vi "Cannon Logic.vi"() -> ()   [LabVIEW 2019]
uses:
  <vilib>/Rock Robotics/WPI/Solenoid/WPI_SolenoidValue.ctl
  <vilib>/Rock Robotics/WPI/ThirdParty/Phoenix-LabVIEW/Motor Controller/Controls/CTRE_Phoenix_MotorControl_ControlMode.ctl
  <vilib>/Rock Robotics/Network Tables/NT Read Boolean.vi
  Robot Global Data.vi
  <vilib>/Rock Robotics/WPI/Solenoid/WPI_SolenoidSetEnum.vi
panel:
  out "ballcount":i16
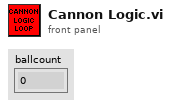
[diagram p1: front panel]
types:
  T1 = typedef "WPI_SolenoidDevRef.ctl" = cluster{"DevStatus":errorcluster, "Pneumatics Control Module":u8, "Forward Solenoid Channel":T2, "Reverse Solenoid Channel":T2}
  T2 = typedef "WPI_SolenoidChannel.ctl" = enum8{"Solenoid 0", "Solenoid 1", "Solenoid 2", "Solenoid 3", "Solenoid 4", "Solenoid 5", "Solenoid 6", "Solenoid 7", "Invalid"}
  T3 = typedef "WPI_MotorControlDeviceRef.ctl" = cluster{"DeviceStatus":errorcluster, "Type":T4, "PWM":cluster{"PWM Channel":T5, "DeadBand":T6}, "CAN":cluster{"Device Number":u8, "SetOutput VI Ref":variant, "GetOutput VI Ref":variant, "Enable VI Ref":variant, "Disable VI Ref":variant, "Data":variant}, "Invert":bool, "DIO PWM":cluster{"PWM \"Enable\" Channel":T5, "DIOChannel":T7, "PWM Rate":dbl}}
  T4 = typedef "WPI_MotorControlType.ctl" = enum16{"PWM", "CAN", "DIO PWM"}
  T5 = typedef "FPGA_DIOPWMChannel.ctl" = enum8{"PWM 0", "PWM 1", "PWM 2", "PWM 3", "PWM 4", "PWM 5", "PWM 6", "PWM 7", "PWM 8", "PWM 9", "PWM MXP 0", "PWM MXP 1", "PWM MXP 2", "PWM MXP 3", "PWM MXP 4", "PWM MXP 5", "PWM MXP 6", "PWM MXP 7", "PWM MXP 8", "PWM MXP 9", "Invalid"}
  T6 = typedef "WPI_PWMDeadband.ctl" = cluster{"Name":string, "maxPositivePwm":i32, "minPositivePwm":i32, "centerPwm":i32, "maxNegativePwm":i32, "minNegativePwm":i32, "angularRange":u16}
  T7 = typedef "FPGA_DIOChannel.ctl" = enum8{"DIO 0", "DIO 1", "DIO 2", "DIO 3", "DIO 4", "DIO 5", "DIO 6", "DIO 7", "DIO 8", "DIO 9", "DIO MXP 0", "DIO MXP 1", "DIO MXP 2", "DIO MXP 3", "DIO MXP 4", "DIO MXP 5", "DIO MXP 6", "DIO MXP 7", "DIO MXP 8", "DIO MXP 9", "DIO MXP 10", "DIO MXP 11", "DIO MXP 12", "DIO MXP 13", "DIO MXP 14", "DIO MXP 15", "SPI Port CS1", "SPI Port CS2", "SPI Port CS3", "SPI Port MISO", "SPI Port MOSI", "Invalid"}
  T8 = typedef "WPI_AnalogChannelDevRef.ctl" = cluster{"DevStatus":errorcluster, "Analog Channel":T9}
  T9 = typedef "FPGA_AIChannel.ctl" = enum8{"AI 0", "AI 1", "AI 2", "AI 3", "AI MXP 0", "AI MXP 1", "AI MXP 2", "AI MXP 3", "Invalid"}
  T10 = typedef "WPI_SolenoidValue.ctl" = enum16{"Off", "On", "Forward", "Reverse"}
  T11 = typedef "CTRE_Phoenix_MotorControl_ControlMode.ctl" = u16
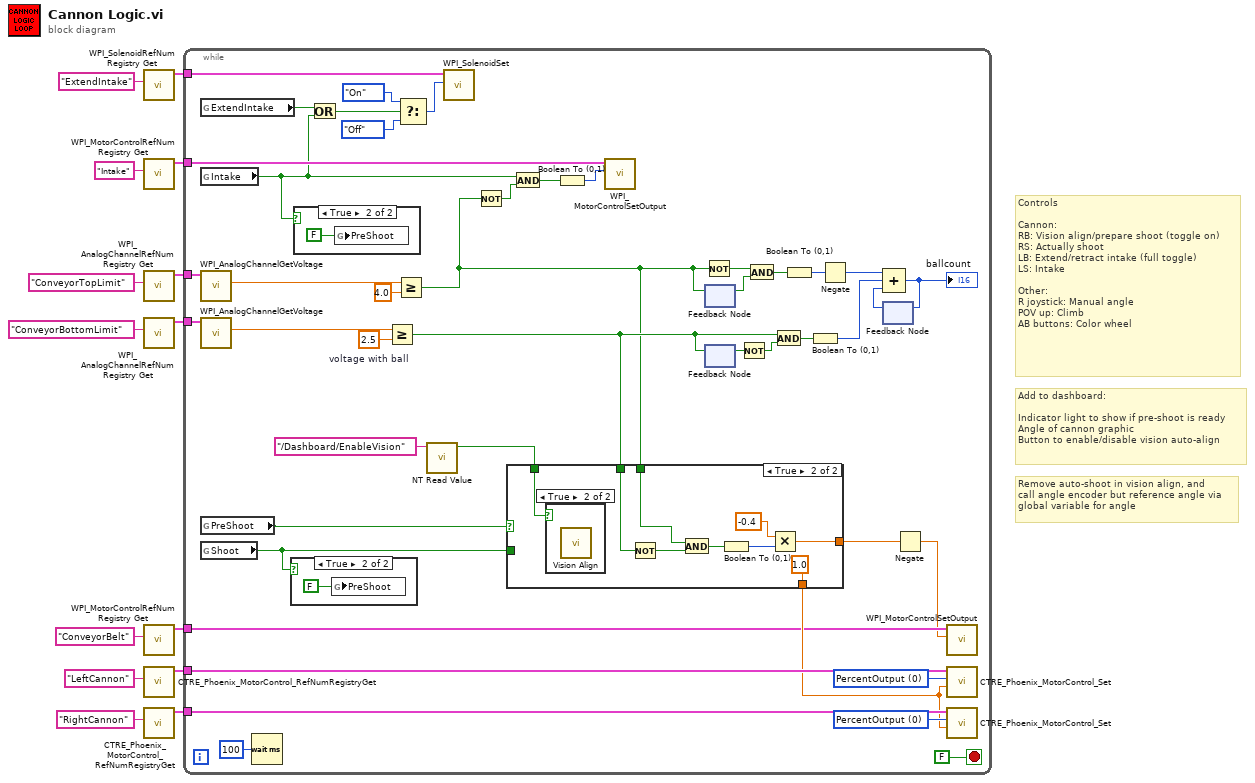
[diagram p0: block diagram]
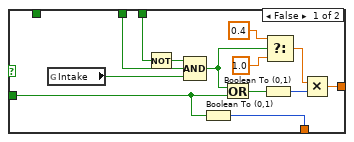
[diagram p4: hidden frame]
diagram:
  # "Remove auto-shoot in vision align, and\ncall angle encoder but reference angle via\nglobal variable for angle"
  # "Add to dashboard:\n\nIndicator light to show if pre-shoot is ready\nAngle of cannon graphic\nButton to enable/disable vision auto-align"
  # "Controls\n\nCannon:\nRB: Vision align/prepare shoot (toggle on)\nRS: Actually shoot\nLB: Extend/retract intake (full toggle)\nLS: Intake\n\nOther:\nR joystick: Manual angle\nPOV up: Climb\nAB buttons: Color wheel"
  n1 = call <vilib>:"WPI_SolenoidRefNum Registry Get.vi"("refnum name"="ExtendIntake") -> ("SolenoidDevRef"=w8:T1)  [unwired: 9 in, 1 out]
  n2 = call <vilib>:"WPI_MotorControlRefNum Registry Get.vi"("refnum name"="Intake") -> ("MotorControlDevRef"=w7:T3)  [unwired: 9 in, 1 out]
  n3 = call <vilib>:"WPI_AnalogChannelRefNum Registry Get.vi"("refnum name"="ConveyorTopLimit") -> ("AIDeviceRef"=w4:T8)  [unwired: 9 in, 1 out]
  n4 = call <vilib>:"WPI_AnalogChannelRefNum Registry Get.vi"("refnum name"="ConveyorBottomLimit") -> ("AIDeviceRef"=w5:T8)  [unwired: 9 in, 1 out]
  n5 = call <vilib>:"WPI_MotorControlRefNum Registry Get.vi"("refnum name"="ConveyorBelt") -> ("MotorControlDevRef"=w3:T3)  [unwired: 9 in, 1 out]
  n6 = call <vilib>:"CTRE_Phoenix_MotorControl_RefNumRegistryGet.vi"("refnum name"="LeftCannon") -> ("PhoenixMotorControlDevRef"=w1:T3)  [unwired: 9 in, 1 out]
  n7 = call <vilib>:"CTRE_Phoenix_MotorControl_RefNumRegistryGet.vi"("refnum name"="RightCannon") -> ("PhoenixMotorControlDevRef"=w6:T3)  [unwired: 9 in, 1 out]
  n8 = while {
    tunnel: w8 -> [w54]
    tunnel: w7 -> [w40]
    tunnel: w6 -> [w52]
    tunnel: w5 -> [w51]
    tunnel: w4 -> [w50]
    tunnel: w3 -> [w39]
    tunnel: w1 -> [w46]
    stop <- FALSE stop-if-true
    w47 = T11 0 items=["PercentOutput"=0, "Position"=1, "Velocity"=2, "Current"=3, "Follower"=5, "MotionProfile"=6, "MotionMagic"=7, "MotionProfileArc"=10, "Disabled"=15] ("Control Mode")
    w45 = T11 0 items=["PercentOutput"=0, "Position"=1, "Velocity"=2, "Current"=3, "Follower"=5, "MotionProfile"=6, "MotionMagic"=7, "MotionProfileArc"=10, "Disabled"=15] ("Control Mode")
    w48 = 2.5  # voltage with ball
    n9 = global read "Robot Global Data.vi" "ExtendIntake"() -> (w26:bool)
    n10 = global read "Robot Global Data.vi" "Intake"() -> (w19:bool)
    n11 = call <vilib>:"WPI_AnalogChannelGetVoltage.vi"("AIDeviceRef"=w50) -> ("Voltage"=w21:dbl)  [unwired: 8 in, 2 out]
    n12 = call <vilib>:"WPI_AnalogChannelGetVoltage.vi"("AIDeviceRef"=w51) -> ("Voltage"=w20:dbl)  [unwired: 8 in, 2 out]
    n13 = global read "Robot Global Data.vi" "PreShoot"() -> (w24:bool)
    n14 = global read "Robot Global Data.vi" "Shoot"() -> (w25:bool)
    n15 = Wait (ms)(milliseconds to wait=u32 100) -> ()  [unwired: 1 out]
    n16 = case shown="True" w25 {
      frame False {
      }
      frame True {
        n17 = global write "Robot Global Data.vi" "PreShoot"(FALSE ("PreShoot")) -> ()
      }
    }
    n18 = case shown="True" w19 {
      frame False {
      }
      frame True {
        n19 = global write "Robot Global Data.vi" "PreShoot"(FALSE ("PreShoot")) -> ()
      }
    }
    n20 = Or(x=w26, y=w19) -> (x .or. y?=w57:bool)
    n21 = Greater Or Equal?(x=w20, y=w48) -> (x >= y?=w16:bool)
    n22 = Greater Or Equal?(x=w21, y=4.0) -> (x >= y?=w15:bool)
    n23 = Select(t=WPI_SolenoidValue."On" ("Value"), s=w57, f=WPI_SolenoidValue."Off" ("Value")) -> (s? t:f=w53:T10)
    n24 = call-poly <vilib>:"NT Read Value.vi"("Name"="/Dashboard/EnableVision") -> ("Boolean"=w38:bool)  [unwired: 9 in, 1 out]
    n25 = call-poly <vilib>:"WPI_SolenoidSet.vi"("Value"=w53, "SolenoidDevRef"=w54) -> ()  [unwired: 8 in, 2 out]
    n26 = Not(x=w15) -> (.not. x?=w17:bool)
    n27 = case shown="True" w24 {
      tunnel: [w71 w74] -> w22
      tunnel: [w70 1.0] -> w41
      tunnel: w25 -> [w62 _]
      tunnel: w15 -> [w63 w76]
      tunnel: w38 -> [_ w82]
      tunnel: w16 -> [w72 w77]
      frame False {
        n28 = global read "Robot Global Data.vi" "Intake"() -> (w69:bool)
        n29 = Not(x=w63) -> (.not. x?=w61:bool)
        n30 = Compound Arithmetic op=AND(w61, w72, w69) -> (w67:bool)
        n31 = Boolean To (0,1)(Boolean=w62) -> (0, 1=w70:i16)
        n32 = Or(x=w67, y=w62) -> (x .or. y?=w73:bool)
        n33 = Boolean To (0,1)(Boolean=w73) -> (0, 1=w65:i16)
        n34 = Select(t=0.4, s=w67, f=1.0) -> (s? t:f=w64:dbl)
        n35 = Multiply(x=w64, y=w65) -> (x*y=w71:dbl)
      }
      frame True {
        n36 = case shown="True" w82 {
          frame False {
          }
          frame True {
            n37 = call "Vision Align.vi"() -> ()  [unwired: 12 in]
          }
        }
        n38 = Not(x=w77) -> (.not. x?=w75:bool)
        n39 = And(x=w76, y=w75) -> (x .and. y?=w79:bool)
        n40 = Boolean To (0,1)(Boolean=w79) -> (0, 1=w80:i16)
        n41 = Multiply(x=-0.4, y=w80) -> (x*y=w74:dbl)
      }
    }
    n42 = And(x=w19, y=w17) -> (x .and. y?=w18:bool)
    n43 = Boolean To (0,1)(Boolean=w18) -> (0, 1=w49:i16)
    n44 = call <vilib>:"WPI_MotorControlSetOutput.vi"("Output"=w49, "MotorControlDevRef"=w40) -> ()  [unwired: 7 in, 3 out]
    n45 = Not(x=w15) -> (.not. x?=w37:bool)
    n46 = feedback-in #1(w15) -> ()
    n47 = feedback #1() -> (w36:bool)  [unwired: 1 in]
    n48 = feedback #2() -> (w35:bool)  [unwired: 1 in]
    n49 = feedback-in #2(w16) -> ()
    n50 = Not(x=w35) -> (.not. x?=w34:bool)
    n51 = And(x=w37, y=w36) -> (x .and. y?=w33:bool)
    n52 = And(x=w16, y=w34) -> (x .and. y?=w32:bool)
    n53 = Boolean To (0,1)(Boolean=w33) -> (0, 1=w31:i16)
    n54 = Boolean To (0,1)(Boolean=w32) -> (0, 1=w27:i16)
    n55 = Negate(x=w31) -> (-x=w30:i16)
    n56 = feedback #3() -> (w29:i16)  [unwired: 1 in]
    n57 = Compound Arithmetic op=ADD(w30, w27, w29) -> (w28:i16)
    "ballcount" <- w28
    n58 = feedback-in #3(w28) -> ()
    n59 = Negate(x=w22) -> (-x=w23:dbl)
    n60 = call <vilib>:"WPI_MotorControlSetOutput.vi"("Output"=w23, "MotorControlDevRef"=w39) -> ()  [unwired: 7 in, 3 out]
    n61 = call <vilib>:"CTRE_Phoenix_MotorControl_Set.vi"("Output"=w41, "Control Mode"=w47, "PhoenixMotorControlDevRef"=w46) -> ()  [unwired: 7 in, 2 out]
    n62 = call <vilib>:"CTRE_Phoenix_MotorControl_Set.vi"("Output"=w41, "Control Mode"=w45, "PhoenixMotorControlDevRef"=w52) -> ()  [unwired: 7 in, 2 out]
  }
